vi "读取反控数据解析(子VI).vi"(6 "数据":string, 7 "命令编码CN":string) -> (2 "设置超时时间/min":i32=1, 3 "反控命令错误？":bool)   [LabVIEW 2016, in "数据传输系统-06.lvlib"]
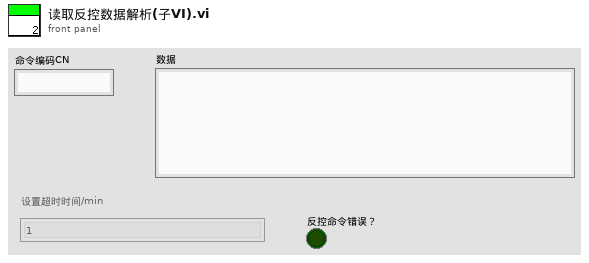
[diagram p1: front panel]
types:
  T1 = typedef "数据传输系统-06.lvlib/应用环境.ctl" = enum16{"STD", "GB212", "婉仪平台"}
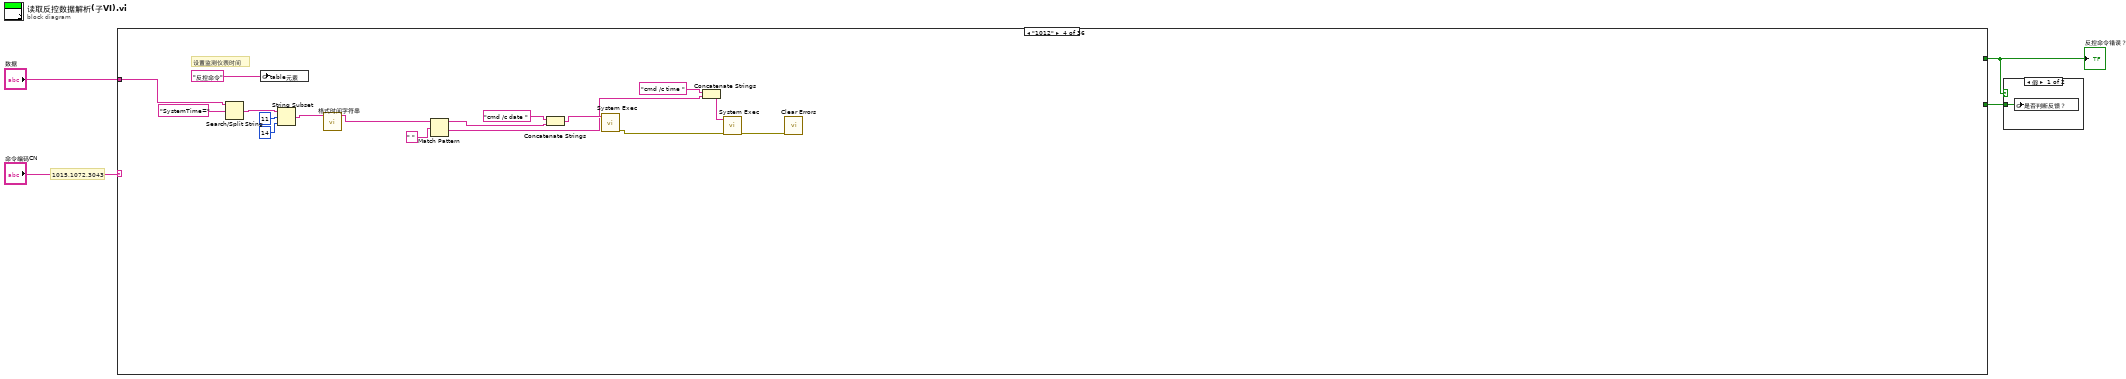
[diagram p0: block diagram]
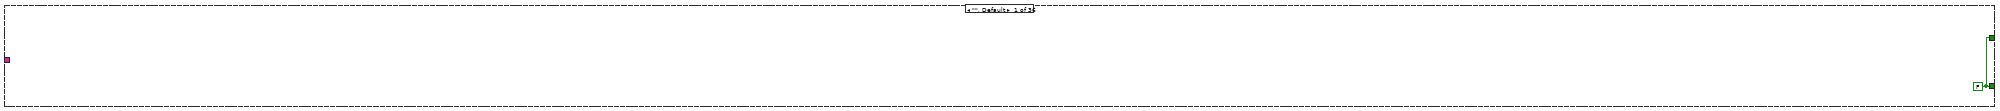
[diagram p2: hidden frame]
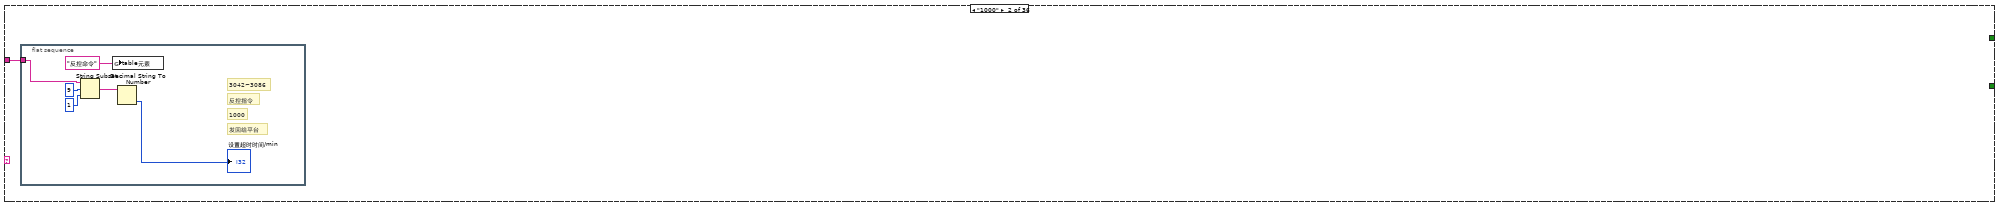
[diagram p3: hidden frame]
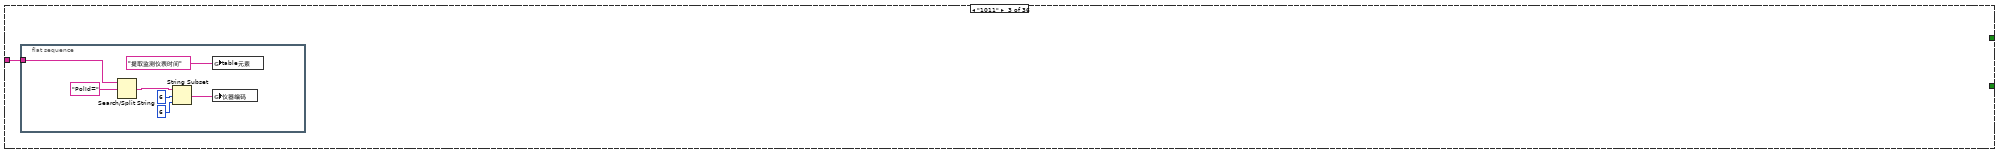
[diagram p4: hidden frame]
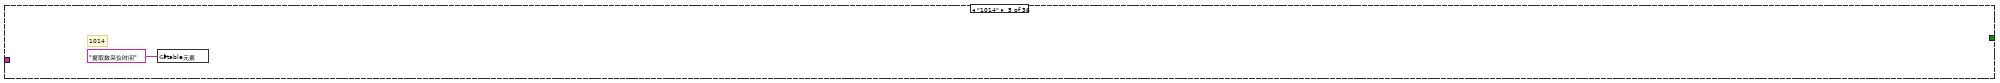
[diagram p5: hidden frame]
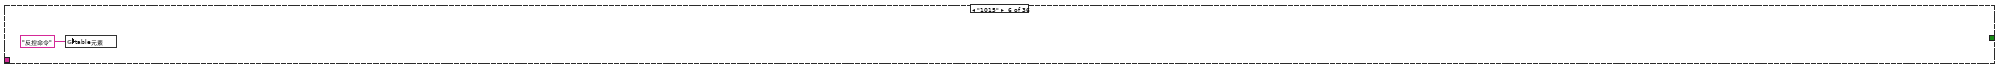
[diagram p6: hidden frame]
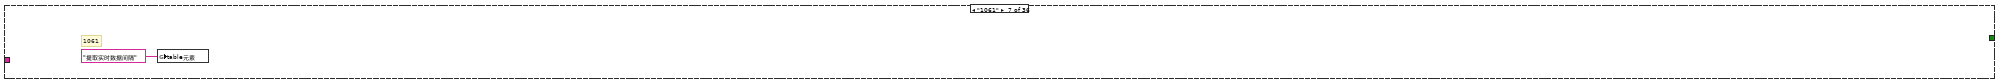
[diagram p7: hidden frame]
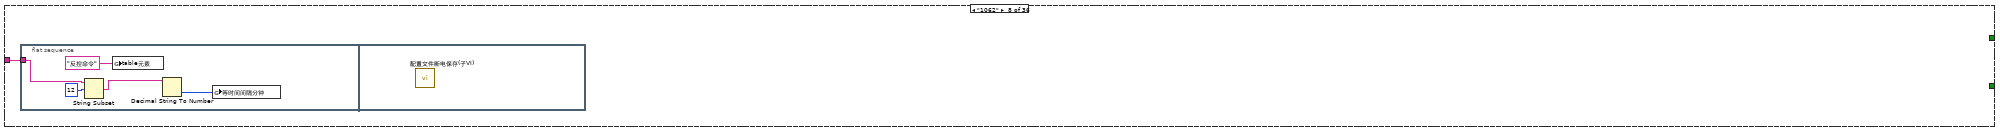
[diagram p8: hidden frame]
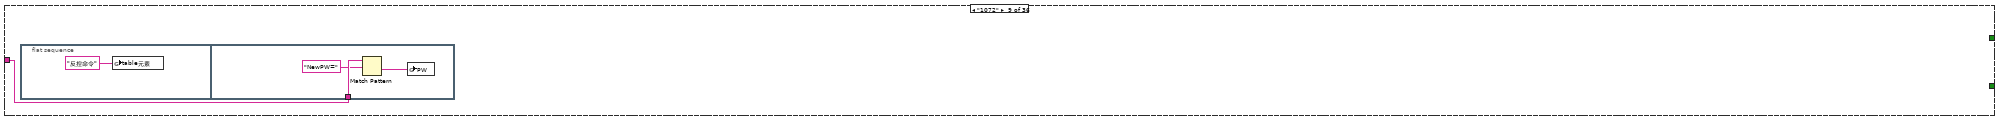
[diagram p9: hidden frame]
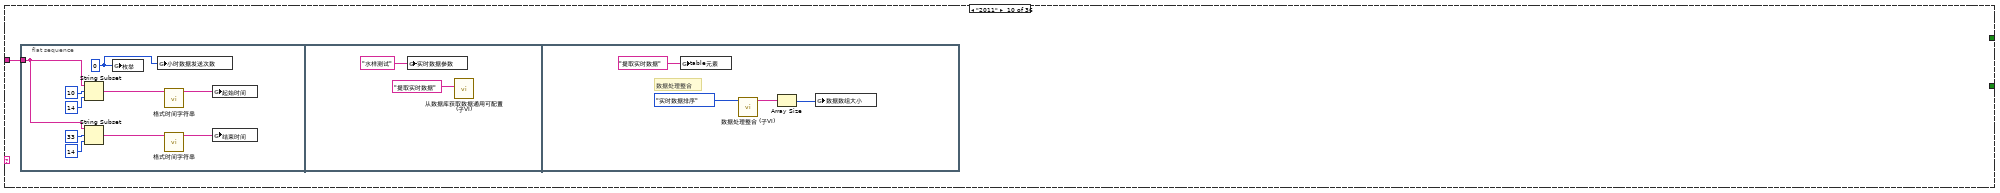
[diagram p10: hidden frame]
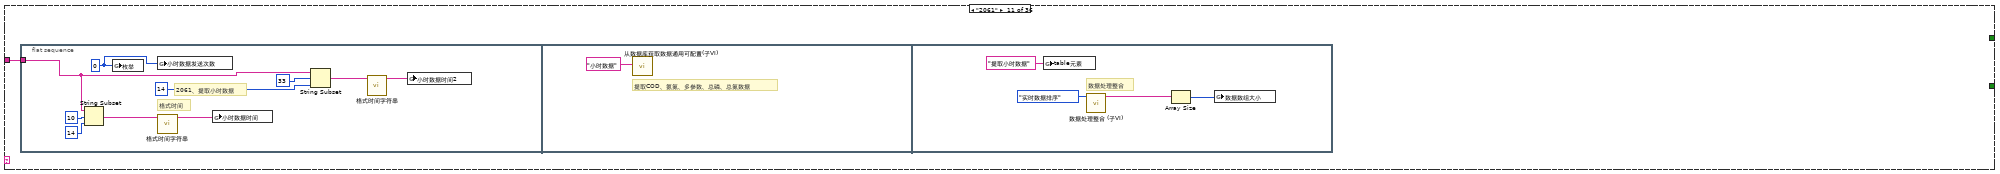
[diagram p11: hidden frame]
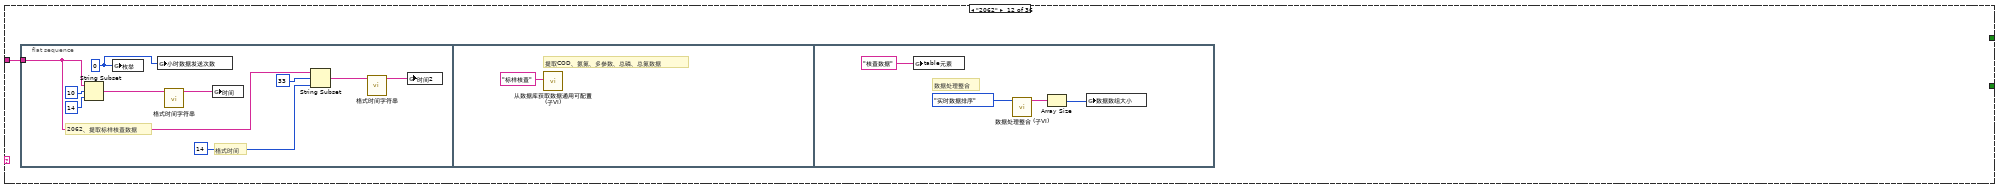
[diagram p12: hidden frame]
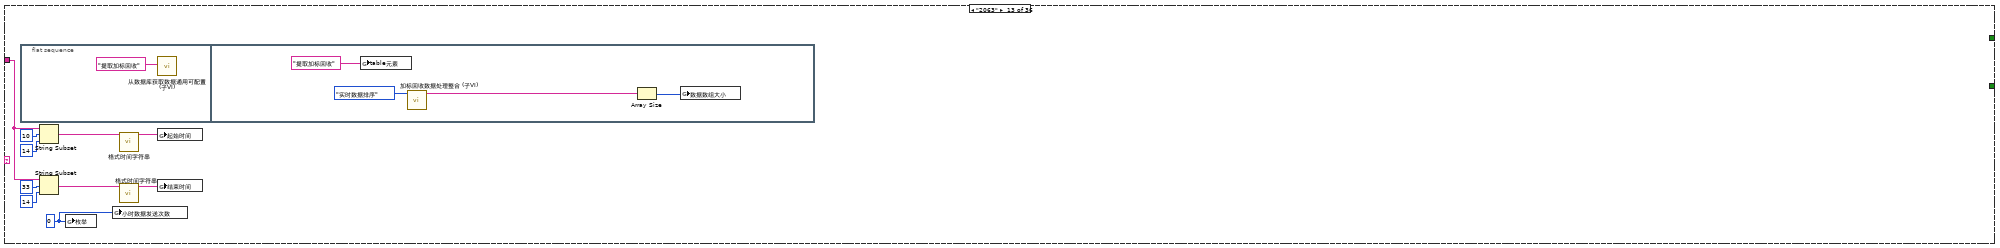
[diagram p13: hidden frame]
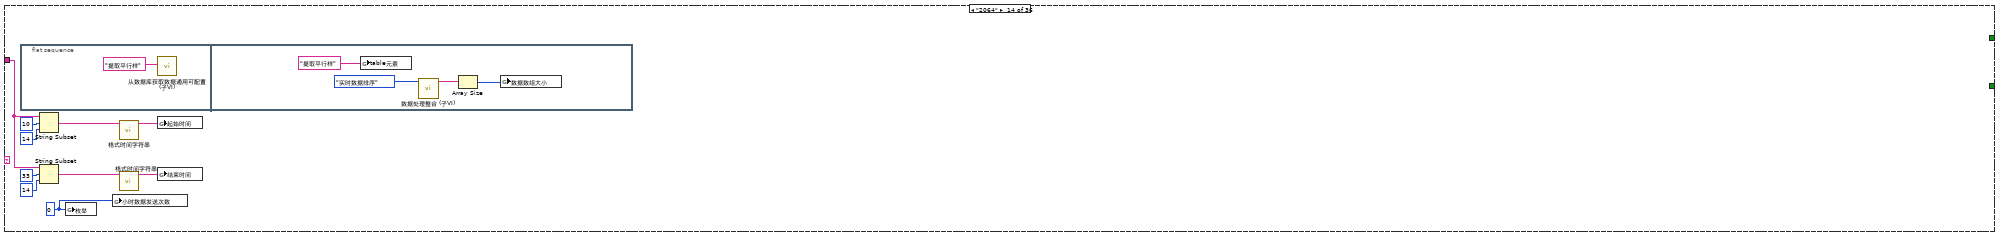
[diagram p14: hidden frame]
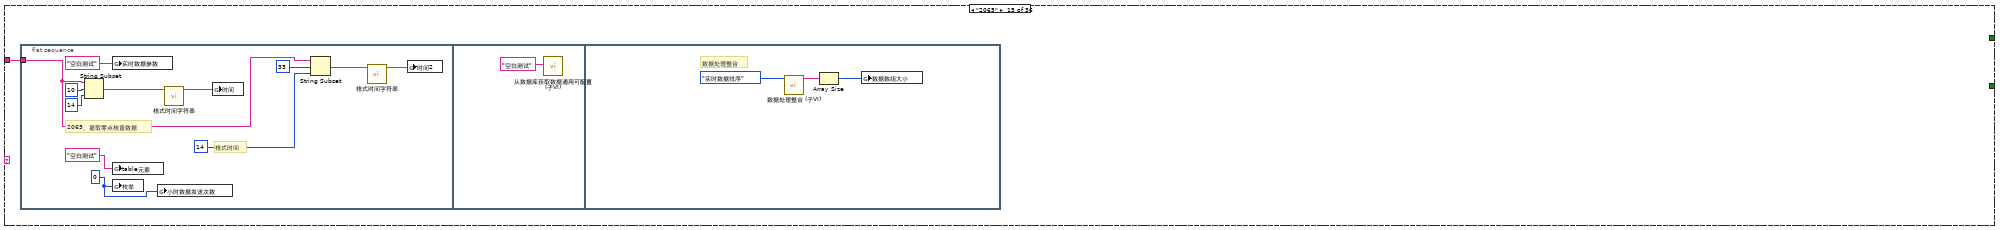
[diagram p15: hidden frame]
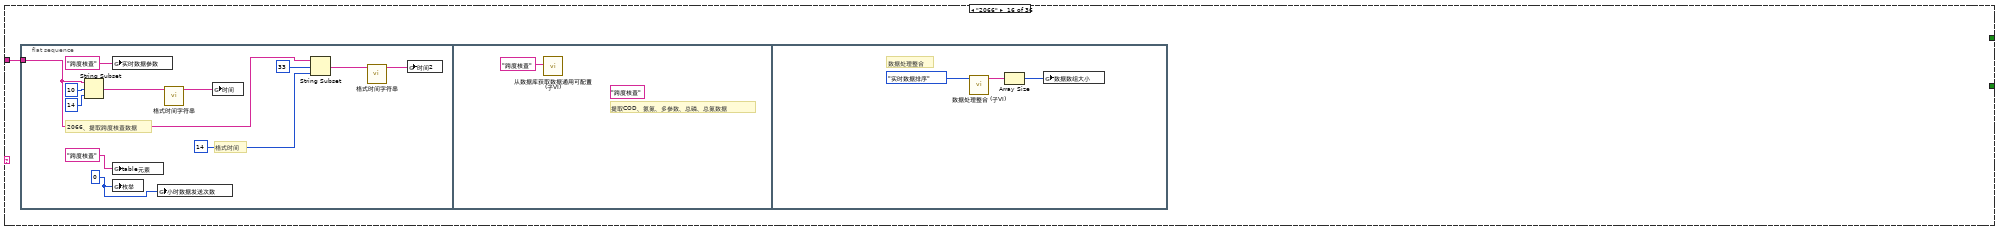
[diagram p16: hidden frame]
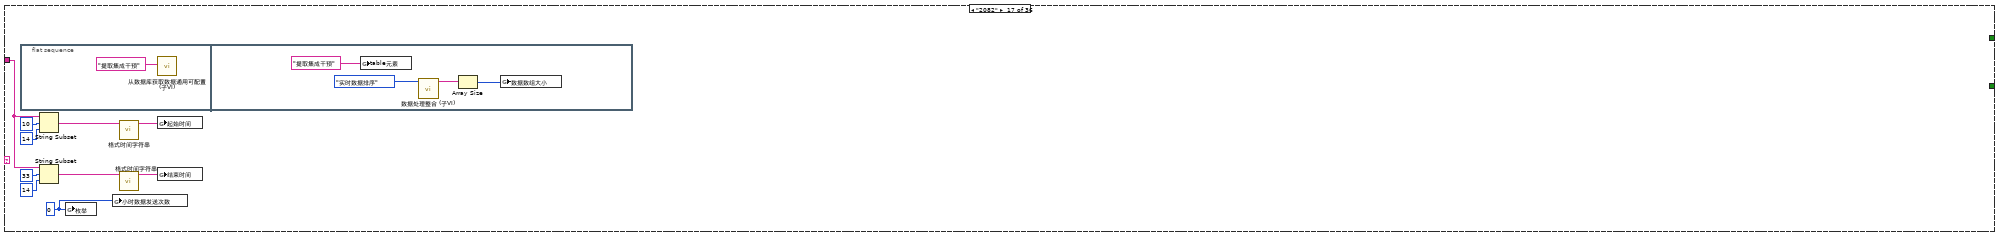
[diagram p17: hidden frame]
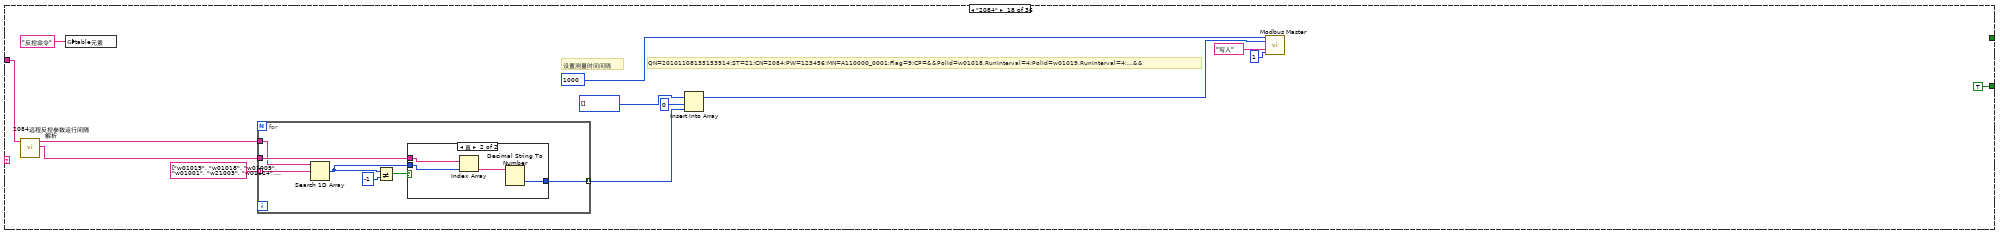
[diagram p18: hidden frame]
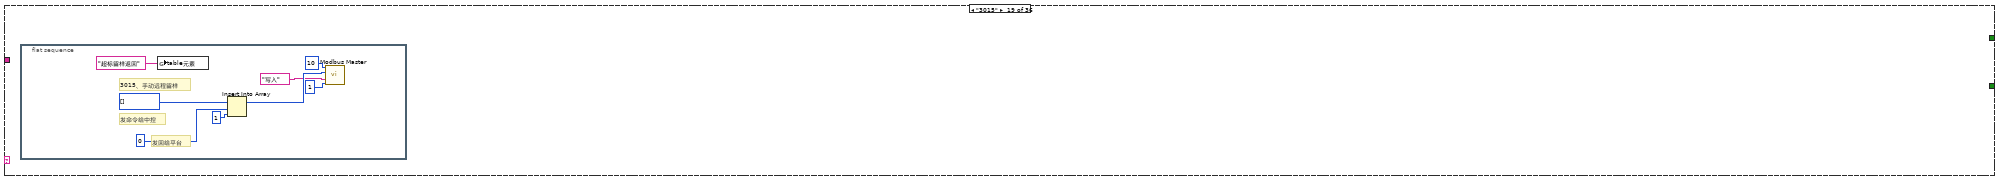
[diagram p20: hidden frame]
diagram:
  # "1015,1072,3043"
  n1 = case shown="\"1012\"" "命令编码CN" {
    selector: "命令编码CN" -> [_ _ _ _ _ _ _ _ _ _ _ _ _ _ _ _ _ _ _ _ _ _ _ _ _ _ _ _ _ w509 _ _ _ _ w649 _]
    tunnel: "数据" -> [_ w6 w13 w32 _ _ _ w41 w47 w52 w69 w85 w102 w116 w131 w148 w165 w191 _ w212 w368 _ _ w460 _ _ _ _ w508 w510 _ w571 w592 w613 w648 _]
    tunnel: [w5 _ _ _ _ _ _ _ _ _ _ _ _ _ _ _ _ _ _ _ _ _ _ _ _ _ _ _ _ _ _ _ _ _ _ _] -> w2
    tunnel: [w5 _ _ _ _ _ _ _ _ _ _ _ _ _ _ _ _ TRUE _ _ TRUE _ _ TRUE ("是否判断反馈？") _ _ _ _ _ TRUE _ _ _ _ _ _] -> w1
    frame "", Default {
      w5 = FALSE
    }
    frame "1000" {
      n2 = flat-sequence {
        tunnel: w6 -> [w8]
        frame #0 {
          # "发回给平台"
          # "3042~3086"
          # "反控指令"
          # "1000"
          n3 = String Subset(string=w8, offset (0)=9 ("偏移量(0)"), length (rest)=1 ("长度（剩余）")) -> (substring=w10:string)
          n4 = global write "全局1.vi" "table元素"("反控命令" ("新元素/子数组")) -> ()
          n5 = Decimal String To Number(string=w10) -> (number=→"设置超时时间/min":i32)  [unwired: 2 in, 1 out]
        }
      }
    }
    frame "1011" {
      n6 = flat-sequence {
        tunnel: w13 -> [w14]
        frame #0 {
          n7 = Search/Split String(string=w14, search string/char (-)="PolId=" ("搜索字符串/字符(-)")) -> (match + rest of string=w19:string)  [unwired: 1 in, 2 out]
          n8 = String Subset(string=w19, offset (0)=6 ("偏移量(0)"), length (rest)=6 ("长度（剩余）")) -> (substring=w16:string)
          n9 = global write "全局1.vi" "table元素"("提取监测仪表时间") -> ()
          n10 = global write "全局 提取仪器参数.vi" "仪器编码"(w16) -> ()
        }
      }
    }
    frame "1012" {
      # "设置监测仪表时间"
      n11 = Search/Split String(string=w32, search string/char (-)="SystemTime=" ("搜索字符串/字符(-)")) -> (match + rest of string=w35:string)  [unwired: 1 in, 2 out]
      n12 = global write "全局1.vi" "table元素"("反控命令" ("新元素/子数组")) -> ()
      n13 = String Subset(string=w35, offset (0)=11 ("偏移量(0)"), length (rest)=14 ("长度（剩余）")) -> (substring=w31:string)
      n14 = call "格式时间字符串.vi"("字符串"=w31) -> ("连接的字符串"=w29:string)  [unwired: 10 in]
      n15 = Match Pattern(string=w29, regular expression=" " ("子字符串;substring")) -> (before substring=w27:string, after substring=w23:string)  [unwired: 1 in, 2 out]
      n16 = Concatenate Strings("cmd /c date " ("command line"), w27) -> (w26:string)
      n17 = call <vilib>:"System Exec.vi"("command line"=w26) -> ("error out"=w25:errorcluster)  [unwired: 7 in, 3 out]
      n18 = Concatenate Strings("cmd /c time " ("command line"), w23) -> (w22:string)
      n19 = call <vilib>:"System Exec.vi"("error in (no error)"=w25, "command line"=w22) -> ("error out"=w21:errorcluster)  [unwired: 6 in, 3 out]
      n20 = call <vilib>:"Clear Errors.vi"("error in (no error)"=w21) -> ()  [unwired: 5 in, 2 out]
    }
    frame "1014" {
      # "1014"
      n21 = global write "全局1.vi" "table元素"("提取数采仪时间") -> ()
    }
    frame "1015" {
      n22 = global write "全局1.vi" "table元素"("反控命令" ("新元素/子数组")) -> ()
    }
    frame "1061" {
      # "1061"
      n23 = global write "全局1.vi" "table元素"("提取实时数据间隔") -> ()
    }
    frame "1062" {
      n24 = flat-sequence {
        tunnel: w41 -> [w44]
        frame #0 {
          n25 = String Subset(string=w44, offset (0)=12 ("偏移量(0)")) -> (substring=w45:string)  [unwired: 1 in]
          n26 = global write "全局1.vi" "table元素"("反控命令" ("新元素/子数组")) -> ()
          n27 = Decimal String To Number(string=w45) -> (number=w42:i32)  [unwired: 2 in, 1 out]
          n28 = global write "断电保存全局.vi" "等时间间隔分钟"(w42) -> ()
        }
        frame #1 {
          n29 = call "配置文件断电保存(子VI).vi"() -> ()  [unwired: 12 in]
        }
      }
    }
    frame "1072" {
      n30 = flat-sequence {
        tunnel: w47 -> [w51]
        frame #0 {
          n31 = global write "全局1.vi" "table元素"("反控命令" ("新元素/子数组")) -> ()
        }
        frame #1 {
          n32 = Match Pattern(string=w51, regular expression="NewPW=" ("正则表达式")) -> (after substring=w49:string)  [unwired: 1 in, 3 out]
          n33 = global write "断电保存全局.vi" "PW"(w49) -> ()
        }
      }
    }
    frame "2011" {
      n34 = flat-sequence {
        tunnel: w52 -> [w53]
        frame #0 {
          w58 = 0 ("数值")
          n35 = String Subset(string=w53, offset (0)=10 ("偏移量(0)"), length (rest)=14 ("长度（剩余）")) -> (substring=w61:string)
          n36 = String Subset(string=w53, offset (0)=33 ("偏移量(0)"), length (rest)=14 ("长度（剩余）")) -> (substring=w59:string)
          n37 = global write "全局1.vi" "枚举"(w58) -> ()
          n38 = global write "全局 小时数据发送次数.vi" "小时数据发送次数"(w58) -> ()
          n39 = call "格式时间字符串.vi"("字符串"=w61) -> ("连接的字符串"=w62:string)  [unwired: 10 in]
          n40 = call "格式时间字符串.vi"("字符串"=w59) -> ("连接的字符串"=w60:string)  [unwired: 10 in]
          n41 = global write "起始时间.vi" "起始时间"(w62) -> ()
          n42 = global write "起始时间.vi" "结束时间"(w60) -> ()
        }
        frame #1 {
          n43 = global write "全局 实时数据参数.vi" "实时数据参数"("水样测试") -> ()
          n44 = call "从数据库获取数据通用可配置(子VI).vi"("table输入"="提取实时数据" ("新元素/子数组")) -> ()  [unwired: 9 in, 2 out]
        }
        frame #2 {
          # "数据处理整合"
          n45 = global write "全局1.vi" "table元素"("提取实时数据" ("新元素/子数组")) -> ()
          n46 = call "数据处理整合 (子VI).vi"("枚举"=enum16{"实时数据排序", "小时数据排序"}."实时数据排序") -> ("已排序的数组"=w67:string[])  [unwired: 10 in]
          n47 = Array Size(array=w67) -> (size(s)=w68:i32)
          n48 = global write "全局 数据数组大小.vi" "数据数组大小"(w68) -> ()
        }
      }
    }
    frame "2061" {
      n49 = flat-sequence {
        tunnel: w69 -> [w70]
        frame #0 {
          w71 = 0 ("数值")
          # "格式时间"
          # "2061、提取小时数据"
          n50 = String Subset(string=w70, offset (0)=10 ("偏移量(0)"), length (rest)=14 ("长度（剩余）")) -> (substring=w74:string)
          n51 = global write "全局1.vi" "枚举"(w71) -> ()
          n52 = global write "全局 小时数据发送次数.vi" "小时数据发送次数"(w71) -> ()
          n53 = call "格式时间字符串.vi"("字符串"=w74) -> ("连接的字符串"=w75:string)  [unwired: 10 in]
          n54 = global write "全局 水样时间.vi" "小时数据时间"(w75) -> ()
          n55 = String Subset(string=w70, offset (0)=33 ("偏移量(0)"), length (rest)=14 ("长度（剩余）")) -> (substring=w73:string)
          n56 = call "格式时间字符串.vi"("字符串"=w73) -> ("连接的字符串"=w72:string)  [unwired: 10 in]
          n57 = global write "全局 时间2.vi" "小时数据时间2"(w72) -> ()
        }
        frame #1 {
          # "提取COD、氨氮、多参数、总磷、总氮数据"
          n58 = call "从数据库获取数据通用可配置(子VI).vi"("table输入"="小时数据" ("名称（未命名）")) -> ()  [unwired: 9 in, 2 out]
        }
        frame #2 {
          # "数据处理整合"
          n59 = global write "全局1.vi" "table元素"("提取小时数据" ("新元素/子数组")) -> ()
          n60 = call "数据处理整合 (子VI).vi"("枚举"=enum16{"实时数据排序", "小时数据排序"}."实时数据排序") -> ("已排序的数组"=w84:string[])  [unwired: 10 in]
          n61 = Array Size(array=w84) -> (size(s)=w83:i32)
          n62 = global write "全局 数据数组大小.vi" "数据数组大小"(w83) -> ()
        }
      }
    }
    frame "2062" {
      n63 = flat-sequence {
        tunnel: w85 -> [w86]
        frame #0 {
          w87 = 0 ("数值")
          # "格式时间"
          # "2062、提取标样核查数据"
          n64 = String Subset(string=w86, offset (0)=10 ("偏移量(0)"), length (rest)=14 ("长度（剩余）")) -> (substring=w90:string)
          n65 = global write "全局1.vi" "枚举"(w87) -> ()
          n66 = global write "全局 小时数据发送次数.vi" "小时数据发送次数"(w87) -> ()
          n67 = call "格式时间字符串.vi"("字符串"=w90) -> ("连接的字符串"=w91:string)  [unwired: 10 in]
          n68 = global write "全局 水样时间.vi" "时间"(w91) -> ()
          n69 = String Subset(string=w86, offset (0)=33 ("偏移量(0)"), length (rest)=14 ("长度（剩余）")) -> (substring=w89:string)
          n70 = call "格式时间字符串.vi"("字符串"=w89) -> ("连接的字符串"=w88:string)  [unwired: 10 in]
          n71 = global write "全局 时间2.vi" "时间2"(w88) -> ()
        }
        frame #1 {
          # "提取COD、氨氮、多参数、总磷、总氮数据"
          n72 = call "从数据库获取数据通用可配置(子VI).vi"("table输入"="标样核查" ("新元素/子数组")) -> ()  [unwired: 9 in, 2 out]
        }
        frame #2 {
          # "数据处理整合"
          n73 = global write "全局1.vi" "table元素"("核查数据" ("新元素/子数组")) -> ()
          n74 = call "数据处理整合 (子VI).vi"("枚举"=enum16{"实时数据排序", "小时数据排序"}."实时数据排序") -> ("已排序的数组"=w99:string[])  [unwired: 10 in]
          n75 = Array Size(array=w99) -> (size(s)=w100:i32)
          n76 = global write "全局 数据数组大小.vi" "数据数组大小"(w100) -> ()
        }
      }
    }
    frame "2063" {
      w101 = 0 ("数值")
      n77 = flat-sequence {
        frame #0 {
          n78 = call "从数据库获取数据通用可配置(子VI).vi"("table输入"="提取加标回收" ("新元素/子数组")) -> ()  [unwired: 9 in, 2 out]
        }
        frame #1 {
          n79 = global write "全局1.vi" "table元素"("提取加标回收" ("新元素/子数组")) -> ()
          n80 = call "加标回收数据处理整合 (子VI).vi"("枚举"=enum16{"实时数据排序", "小时数据排序"}."实时数据排序") -> ("已排序的数组"=w113:string[])  [unwired: 10 in]
          n81 = Array Size(array=w113) -> (size(s)=w115:i32)
          n82 = global write "全局 数据数组大小.vi" "数据数组大小"(w115) -> ()
        }
      }
      n83 = String Subset(string=w102, offset (0)=10 ("偏移量(0)"), length (rest)=14 ("长度（剩余）")) -> (substring=w104:string)
      n84 = String Subset(string=w102, offset (0)=33 ("偏移量(0)"), length (rest)=14 ("长度（剩余）")) -> (substring=w106:string)
      n85 = global write "全局1.vi" "枚举"(w101) -> ()
      n86 = global write "全局 小时数据发送次数.vi" "小时数据发送次数"(w101) -> ()
      n87 = call "格式时间字符串.vi"("字符串"=w104) -> ("连接的字符串"=w103:string)  [unwired: 10 in]
      n88 = call "格式时间字符串.vi"("字符串"=w106) -> ("连接的字符串"=w105:string)  [unwired: 10 in]
      n89 = global write "起始时间.vi" "起始时间"(w103) -> ()
      n90 = global write "起始时间.vi" "结束时间"(w105) -> ()
    }
    frame "2064" {
      w121 = 0 ("数值")
      n91 = flat-sequence {
        frame #0 {
          n92 = call "从数据库获取数据通用可配置(子VI).vi"("table输入"="提取平行样" ("新元素/子数组")) -> ()  [unwired: 9 in, 2 out]
        }
        frame #1 {
          n93 = global write "全局1.vi" "table元素"("提取平行样" ("新元素/子数组")) -> ()
          n94 = call "数据处理整合 (子VI).vi"("枚举"=enum16{"实时数据排序", "小时数据排序"}."实时数据排序") -> ("已排序的数组"=w130:string[])  [unwired: 10 in]
          n95 = Array Size(array=w130) -> (size(s)=w129:i32)
          n96 = global write "全局 数据数组大小.vi" "数据数组大小"(w129) -> ()
        }
      }
      n97 = String Subset(string=w116, offset (0)=10 ("偏移量(0)"), length (rest)=14 ("长度（剩余）")) -> (substring=w124:string)
      n98 = String Subset(string=w116, offset (0)=33 ("偏移量(0)"), length (rest)=14 ("长度（剩余）")) -> (substring=w122:string)
      n99 = global write "全局1.vi" "枚举"(w121) -> ()
      n100 = global write "全局 小时数据发送次数.vi" "小时数据发送次数"(w121) -> ()
      n101 = call "格式时间字符串.vi"("字符串"=w124) -> ("连接的字符串"=w125:string)  [unwired: 10 in]
      n102 = call "格式时间字符串.vi"("字符串"=w122) -> ("连接的字符串"=w123:string)  [unwired: 10 in]
      n103 = global write "起始时间.vi" "起始时间"(w125) -> ()
      n104 = global write "起始时间.vi" "结束时间"(w123) -> ()
    }
    frame "2065" {
      n105 = flat-sequence {
        tunnel: w131 -> [w133]
        frame #0 {
          w134 = 0 ("数值")
          # "格式时间"
          # "2065、提取零点核查数据"
          n106 = String Subset(string=w133, offset (0)=10 ("偏移量(0)"), length (rest)=14 ("长度（剩余）")) -> (substring=w138:string)
          n107 = global write "全局 实时数据参数.vi" "实时数据参数"("空白测试" ("新元素/子数组")) -> ()
          n108 = global write "全局1.vi" "table元素"("空白测试" ("新元素/子数组")) -> ()
          n109 = global write "全局1.vi" "枚举"(w134) -> ()
          n110 = global write "全局 小时数据发送次数.vi" "小时数据发送次数"(w134) -> ()
          n111 = call "格式时间字符串.vi"("字符串"=w138) -> ("连接的字符串"=w139:string)  [unwired: 10 in]
          n112 = global write "全局 水样时间.vi" "时间"(w139) -> ()
          n113 = String Subset(string=w133, offset (0)=33 ("偏移量(0)"), length (rest)=14 ("长度（剩余）")) -> (substring=w137:string)
          n114 = call "格式时间字符串.vi"("字符串"=w137) -> ("连接的字符串"=w136:string)  [unwired: 10 in]
          n115 = global write "全局 时间2.vi" "时间2"(w136) -> ()
        }
        frame #1 {
          n116 = call "从数据库获取数据通用可配置(子VI).vi"("table输入"="空白测试" ("新元素/子数组")) -> ()  [unwired: 9 in, 2 out]
        }
        frame #2 {
          # "数据处理整合"
          n117 = call "数据处理整合 (子VI).vi"("枚举"=enum16{"实时数据排序", "小时数据排序"}."实时数据排序") -> ("已排序的数组"=w146:string[])  [unwired: 10 in]
          n118 = Array Size(array=w146) -> (size(s)=w147:i32)
          n119 = global write "全局 数据数组大小.vi" "数据数组大小"(w147) -> ()
        }
      }
    }
    frame "2066" {
      n120 = flat-sequence {
        tunnel: w148 -> [w150]
        frame #0 {
          w151 = 0 ("数值")
          # "格式时间"
          # "2066、提取跨度核查数据"
          n121 = String Subset(string=w150, offset (0)=10 ("偏移量(0)"), length (rest)=14 ("长度（剩余）")) -> (substring=w155:string)
          n122 = global write "全局 实时数据参数.vi" "实时数据参数"("跨度核查" ("新元素/子数组")) -> ()
          n123 = global write "全局1.vi" "table元素"("跨度核查" ("新元素/子数组")) -> ()
          n124 = global write "全局1.vi" "枚举"(w151) -> ()
          n125 = global write "全局 小时数据发送次数.vi" "小时数据发送次数"(w151) -> ()
          n126 = call "格式时间字符串.vi"("字符串"=w155) -> ("连接的字符串"=w156:string)  [unwired: 10 in]
          n127 = global write "全局 水样时间.vi" "时间"(w156) -> ()
          n128 = String Subset(string=w150, offset (0)=33 ("偏移量(0)"), length (rest)=14 ("长度（剩余）")) -> (substring=w154:string)
          n129 = call "格式时间字符串.vi"("字符串"=w154) -> ("连接的字符串"=w153:string)  [unwired: 10 in]
          n130 = global write "全局 时间2.vi" "时间2"(w153) -> ()
        }
        frame #1 {
          (unwired) "跨度核查" ("名称（未命名）")
          # "提取COD、氨氮、多参数、总磷、总氮数据"
          n131 = call "从数据库获取数据通用可配置(子VI).vi"("table输入"="跨度核查" ("新元素/子数组")) -> ()  [unwired: 9 in, 2 out]
        }
        frame #2 {
          # "数据处理整合"
          n132 = call "数据处理整合 (子VI).vi"("枚举"=enum16{"实时数据排序", "小时数据排序"}."实时数据排序") -> ("已排序的数组"=w164:string[])  [unwired: 10 in]
          n133 = Array Size(array=w164) -> (size(s)=w163:i32)
          n134 = global write "全局 数据数组大小.vi" "数据数组大小"(w163) -> ()
        }
      }
    }
    frame "2082" {
      w170 = 0 ("数值")
      n135 = flat-sequence {
        frame #0 {
          n136 = call "从数据库获取数据通用可配置(子VI).vi"("table输入"="提取集成干预" ("新元素/子数组")) -> ()  [unwired: 9 in, 2 out]
        }
        frame #1 {
          n137 = global write "全局1.vi" "table元素"("提取集成干预" ("新元素/子数组")) -> ()
          n138 = call "数据处理整合 (子VI).vi"("枚举"=enum16{"实时数据排序", "小时数据排序"}."实时数据排序") -> ("已排序的数组"=w179:string[])  [unwired: 10 in]
          n139 = Array Size(array=w179) -> (size(s)=w178:i32)
          n140 = global write "全局 数据数组大小.vi" "数据数组大小"(w178) -> ()
        }
      }
      n141 = String Subset(string=w165, offset (0)=10 ("偏移量(0)"), length (rest)=14 ("长度（剩余）")) -> (substring=w173:string)
      n142 = String Subset(string=w165, offset (0)=33 ("偏移量(0)"), length (rest)=14 ("长度（剩余）")) -> (substring=w171:string)
      n143 = global write "全局1.vi" "枚举"(w170) -> ()
      n144 = global write "全局 小时数据发送次数.vi" "小时数据发送次数"(w170) -> ()
      n145 = call "格式时间字符串.vi"("字符串"=w173) -> ("连接的字符串"=w174:string)  [unwired: 10 in]
      n146 = call "格式时间字符串.vi"("字符串"=w171) -> ("连接的字符串"=w172:string)  [unwired: 10 in]
      n147 = global write "起始时间.vi" "起始时间"(w174) -> ()
      n148 = global write "起始时间.vi" "结束时间"(w172) -> ()
    }
    frame "2084" {
      # "设置测量时间间隔"
      # "QN=20101108135153914;ST=21;CN=2084;PW=123456;MN=A110000_0001;Flag=9;CP=&&PolId=w01018,RunInterval=4;PolId=w01019,RunInterval=4;...&&"
      n149 = call "2084远程反控参数运行间隔解析.vi"("字符串"=w191) -> ("Value"=w182:string[], "因子编码"=w183:string[])  [unwired: 9 in]
      n150 = global write "全局1.vi" "table元素"("反控命令" ("新元素/子数组")) -> ()
      n151 = for {
        tunnel: w183 -> [w198]
        tunnel: w182 -> [w199]
        tunnel: string[] ["w01019", "w01018", "w01009", "w01001", "w21003", "w01014", "w01010", "w01003", "w21001", "w21011", "w01016", "w19011", "w21006", "w21019", "w01100", "w20120", "w20115", "w20122", "w20123", "w20121", "w20124", "w20111"] ("因子编码") -> [w197] mode=indexing
        tunnel: [w193] -> w181 mode=indexing
        n152 = Search 1D Array(1D array=w198, element=w197) -> (index of element=w194:i32)  [unwired: 1 in]
        n153 = Not Equal?(x=w194, y=-1) -> (x != y?=w195:bool)
        n154 = case shown="真" w195 {
          tunnel: w199 -> [_ w203]
          tunnel: w194 -> [_ w202]
          tunnel: [_ w200] -> w193
          frame False {
          }
          frame True {
            n155 = Index Array(array=w203, index=w202) -> (element=w201:string)
            n156 = Decimal String To Number(string=w201) -> (number=w200:i32)  [unwired: 2 in, 1 out]
          }
        }
      }
      n157 = Insert Into Array(array=u16[] [] ("holding register values"), index=0 ("索引"), new element=w181) -> (w187:u16[])
      n158 = call "Modbus Master.vi"("starting address"=u16 1000, "holding register values"=w187, "读取写入选择"="写入", "Unit ID"=u8 1) -> ()  [unwired: 5 in, 7 out]
    }
    frame "3015" {
      n159 = flat-sequence {
        frame #0 {
          # "发命令给中控"
          # "发回给平台"
          # "3015、手动远程留样"
          n160 = global write "全局1.vi" "table元素"("超标留样返回" ("新元素/子数组")) -> ()
          n161 = Insert Into Array(array=u16[] [] ("holding register values"), index=0 ("索引"), new element=u16 1 ("新元素/子数组")) -> (w207:u16[])
          n162 = call "Modbus Master.vi"("starting address"=u16 10, "holding register values"=w207, "读取写入选择"="写入", "Unit ID"=u8 1) -> ()  [unwired: 5 in, 7 out]
        }
      }
    }
    frame "3020" {
      n163 = flat-sequence {
        tunnel: [w224] -> w218
        tunnel: [w225] -> w217
        tunnel: [w221] -> w216
        tunnel: [w223] -> w215
        tunnel: w212 -> [w222]
        tunnel: [w222] -> w214
        tunnel: w218 -> [w253]
        tunnel: w217 -> [w254]
        tunnel: w216 -> [w255]
        tunnel: w215 -> [w257]
        tunnel: [w256] -> w213
        tunnel: w214 -> [w256]
        tunnel: w213 -> [w340]
        frame #0 {
          w219 = "操作日志报警信息" ("名称（未命名）")
          w228 = 0 ("数值")
          # "3020、提取日志、报警，仪器参数"
          n164 = call "日志报警参数选择 (子VI).vi"("String输入"=w222) -> ("输出boll数组"=w220:bool[], "输出char数组"=w221:string[])  [unwired: 7 in, 2 out]
          n165 = global write "全局1.vi" "枚举"(w228) -> ()
          n166 = global write "全局 小时数据发送次数.vi" "小时数据发送次数"(w228) -> ()
          n167 = Search/Split String(string=w222, search string/char (-)="BeginTime=" ("搜索字符串")) -> (match + rest of string=w227:string)  [unwired: 1 in, 2 out]
          n168 = case shown="\"\"" w227 {
            tunnel: ["1904/01/01 00:00:00" w250] -> w230
            tunnel: w227 -> [_ w244]
            tunnel: [w238 w245] -> w226
            frame "" {
              n169 = Get Date/Time In Seconds() -> (seconds since 1Jan1904=w240:timestamp)
              n170 = Format Date/Time String(time format string (%c)="%Y/%m/%d %H:%M:%S" ("时间格式字符串(%c)"), seconds (now)=w240) -> (date/time string=w241:string)  [unwired: 1 in]
              n171 = Search and Replace String(input string=w241, search string="." ("搜索字符串")) -> (result string=w238:string)  [unwired: 6 in, 3 out]
            }
            frame "真", Default {
              # "格式时间"
              n172 = String Subset(string=w244, offset (0)=10 ("偏移量(0)"), length (rest)=14 ("长度（剩余）")) -> (substring=w249:string)
              n173 = String Subset(string=w244, offset (0)=33 ("偏移量(0)"), length (rest)=14 ("长度（剩余）")) -> (substring=w248:string)
              n174 = call "格式时间字符串.vi"("字符串"=w249) -> ("连接的字符串"=w250:string)  [unwired: 10 in]
              n175 = call "格式时间字符串.vi"("字符串"=w248) -> ("连接的字符串"=w245:string)  [unwired: 10 in]
            }
          }
          n176 = Or Array Elements(Boolean array=w220) -> (logical OR=w223:bool)
          n177 = Obtain Queue(name (unnamed)=w219, element data type=w219) -> (queue out=w224:refnum<queue>, error out=w225:errorcluster)  [unwired: 3 in, 1 out]
          n178 = case shown="真" w223 {
            tunnel: w224 -> [_ w232]
            tunnel: w220 -> [_ w231]
            frame False {
            }
            frame True {
              n179 = for {
                tunnel: w231 -> [w234] mode=indexing
                tunnel: w232 -> [w233]
                i -> [w235]
                n180 = case shown="真" w234 {
                  tunnel: w235 -> [_ w237]
                  tunnel: w233 -> [_ w236]
                  frame False {
                  }
                  frame True {
                    n181 = call "提取日志报警参数入列队 (子VI).vi"("索引"=w237, "队列输入"=w236) -> ()  [unwired: 10 in]
                  }
                }
              }
            }
          }
          n182 = global write "全局 水样时间.vi" "时间"(w230) -> ()
          n183 = global write "全局 时间2.vi" "时间2"(w226) -> ()
        }
        frame #1 {
          # "按需求提取COD、氨氮、总磷、总氮日志"
          # "按需求提取COD、氨氮、总磷、总氮日志"
          n184 = case shown="真" w257 {
            tunnel: w254 -> [_ w260]
            tunnel: w253 -> [_ w259]
            tunnel: w255 -> [_ w258]
            frame False {
            }
            frame True {
              n185 = while {
                shift-right: [w261] -> _
                shift-left: w259 -> [w268]
                tunnel: w260 -> [w267]
                tunnel: w258 -> [w262]
                stop <- w264 stop-if-true
                n186 = Dequeue Element(queue=w268, error in (no error)=w267) -> (queue out=w266:refnum<queue>, element=w263:string)  [unwired: 1 in, 2 out]
                n187 = case shown="\"CODMn\", 默认" w263 {
                  tunnel: w266 -> [_ _ _ _ _ _ _ _ _ _ _ _ _ _]
                  tunnel: w262 -> [w270 w275 w280 w285 w290 w296 w299 w304 w309 w314 w319 w324 w329 w334]
                  frame "CODMn", Default {
                    n188 = Index Array(array=w270, index=0 ("索引")) -> (element=w269:string)
                    n189 = call "数据表比对.vi"("仪器日志参数"="CODMn" ("元素"), "table输入"=w269) -> ("待发送数据"=w272:string[][])  [unwired: 6 in, 3 out]
                    n190 = global write "全局 所有参数.vi" "CODMn"(w272) -> ()
                  }
                  frame "CODCr" {
                    n191 = Index Array(array=w275, index=1 ("索引")) -> (element=w274:string)
                    n192 = call "数据表比对.vi"("仪器日志参数"="CODCr" ("元素"), "table输入"=w274) -> ("待发送数据"=w277:string[][])  [unwired: 6 in, 3 out]
                    n193 = global write "全局 所有参数.vi" "CODCr"(w277) -> ()
                  }
                  frame "氨氮" {
                    n194 = Index Array(array=w280, index=2 ("索引")) -> (element=w279:string)
                    n195 = call "数据表比对.vi"("仪器日志参数"="氨氮" ("元素"), "table输入"=w279) -> ("待发送数据"=w282:string[][])  [unwired: 6 in, 3 out]
                    n196 = global write "全局 所有参数.vi" "氨氮"(w282) -> ()
                  }
                  frame "总磷" {
                    n197 = Index Array(array=w285, index=3 ("索引")) -> (element=w284:string)
                    n198 = call "数据表比对.vi"("仪器日志参数"="总磷" ("元素"), "table输入"=w284) -> ("待发送数据"=w287:string[][])  [unwired: 6 in, 3 out]
                    n199 = global write "全局 所有参数.vi" "总磷"(w287) -> ()
                  }
                  frame "总氮" {
                    n200 = Index Array(array=w290, index=4 ("索引")) -> (element=w289:string)
                    n201 = call "数据表比对.vi"("仪器日志参数"="总氮" ("元素"), "table输入"=w289) -> ("待发送数据"=w292:string[][])  [unwired: 6 in, 3 out]
                    n202 = global write "全局 所有参数.vi" "总氮"(w292) -> ()
                  }
                  frame "数采仪" {
                    n203 = Index Array(array=w296, index=5 ("索引")) -> (element=w294:string)
                    n204 = call "数据表比对.vi"("仪器日志参数"="系统" ("元素"), "table输入"=w294) -> ("待发送数据"=w297:string[][])  [unwired: 6 in, 3 out]
                    n205 = global write "全局 所有参数.vi" "DO"(w297) -> ()
                  }
                  frame "PH" {
                    n206 = Index Array(array=w299, index=6 ("索引")) -> (element=w300:string)
                    n207 = call "数据表比对.vi"("仪器日志参数"="PH" ("元素"), "table输入"=w300) -> ("待发送数据"=w302:string[][])  [unwired: 6 in, 3 out]
                    n208 = global write "全局 所有参数.vi" "PH"(w302) -> ()
                  }
                  frame "电导率" {
                    n209 = Index Array(array=w304, index=7 ("索引")) -> (element=w305:string)
                    n210 = call "数据表比对.vi"("仪器日志参数"="电导率" ("元素"), "table输入"=w305) -> ("待发送数据"=w307:string[][])  [unwired: 6 in, 3 out]
                    n211 = global write "全局 所有参数.vi" "电导率"(w307) -> ()
                  }
                  frame "水温" {
                    n212 = Index Array(array=w309, index=8 ("索引")) -> (element=w310:string)
                    n213 = call "数据表比对.vi"("仪器日志参数"="水温" ("元素"), "table输入"=w310) -> ("待发送数据"=w312:string[][])  [unwired: 6 in, 3 out]
                    n214 = global write "全局 所有参数.vi" "水温"(w312) -> ()
                  }
                  frame "DO" {
                    n215 = Index Array(array=w314, index=9 ("索引")) -> (element=w315:string)
                    n216 = call "数据表比对.vi"("仪器日志参数"="溶解氧" ("元素"), "table输入"=w315) -> ("待发送数据"=w317:string[][])  [unwired: 6 in, 3 out]
                    n217 = global write "全局 所有参数.vi" "DO"(w317) -> ()
                  }
                  frame "浊度" {
                    n218 = Index Array(array=w319, index=10 ("索引")) -> (element=w320:string)
                    n219 = call "数据表比对.vi"("仪器日志参数"="浊度" ("元素"), "table输入"=w320) -> ("待发送数据"=w322:string[][])  [unwired: 6 in, 3 out]
                    n220 = global write "全局 所有参数.vi" "浊度"(w322) -> ()
                  }
                  frame "叶绿素" {
                    n221 = Index Array(array=w324, index=11 ("索引")) -> (element=w325:string)
                    n222 = call "数据表比对.vi"("仪器日志参数"="叶绿素" ("元素"), "table输入"=w325) -> ("待发送数据"=w327:string[][])  [unwired: 6 in, 3 out]
                    n223 = global write "全局 所有参数.vi" "叶绿素"(w327) -> ()
                  }
                  frame "藻密度" {
                    n224 = Index Array(array=w329, index=12 ("索引")) -> (element=w330:string)
                    n225 = call "数据表比对.vi"("仪器日志参数"="藻密度" ("元素"), "table输入"=w330) -> ("待发送数据"=w332:string[][])  [unwired: 6 in, 3 out]
                    n226 = global write "全局 所有参数.vi" "藻密度"(w332) -> ()
                  }
                  frame "ORP" {
                    n227 = Index Array(array=w334, index=13 ("索引")) -> (element=w335:string)
                    n228 = call "数据表比对.vi"("仪器日志参数"="ORP" ("元素"), "table输入"=w335) -> ("待发送数据"=w337:string[][])  [unwired: 6 in, 3 out]
                    n229 = global write "全局 所有参数.vi" "ORP"(w337) -> ()
                  }
                }
                n230 = Get Queue Status(queue=w266) -> (queue out=w261:refnum<queue>, # elements in queue=w265:i32)  [unwired: 2 in, 6 out]
                n231 = Equal To 0?(x=w265) -> (x = 0?=w264:bool)
              }
            }
          }
        }
        frame #2 {
          w349 = "InfoId=" ("搜索字符串/字符(-)")
          n232 = Spreadsheet String To Array(delimiter (Tab)=";" ("分隔符(Tab)"), format string="" ("格式字符串"), spreadsheet string=w340, array type (2D Dbl)=string[] []) -> (array=w341:string[])
          n233 = Index Array(array=w341) -> (element=w339:string)  [unwired: 1 in]
          n234 = Search/Split String(string=w339, search string/char (-)=w349) -> (match + rest of string=w348:string)  [unwired: 1 in, 2 out]
          n235 = Search and Replace String(replace all?=TRUE ("替换全部？(F)"), input string=w348, search string=w349, replace string="" ("替换字符串(\"\")")) -> (result string=w345:string)  [unwired: 4 in, 3 out]
          n236 = Spreadsheet String To Array(delimiter (Tab)="," ("分隔符(Tab)"), format string="" ("格式字符串"), spreadsheet string=w345, array type (2D Dbl)=string[] []) -> (array=w347:string[])
          n237 = Index Array(array=w347) -> (element=w346:string)  [unwired: 1 in]
          n238 = case shown="\"i12001\"" w346 {
            tunnel: ["操作日志" ("名称（未命名）") "提取仪器参数" ("名称（未命名）") "报警信息" ("名称（未命名）") "" ("名称（未命名）")] -> w355
            tunnel: [w357 1 ("数据数组大小") 1 _] -> w356
            tunnel: w345 -> [_ w361 _ _]
            frame "i11001", "i21001" {
              # "数据处理整合"
              # "i11001日志"
              n239 = call "数据处理整合 (子VI).vi"("枚举"=enum16{"实时数据排序", "小时数据排序"}."实时数据排序") -> ("已排序的数组"=w358:string[])  [unwired: 10 in]
              n240 = Array Size(array=w358) -> (size(s)=w357:i32)
            }
            frame "i13001", "i13002", "i13003", "i13004", "i13005", "i13006", "i13007", "i13008", "i13009", "i13010", "i13011", "i13012", "i13013", "i13014", "i13015", "i13016", "i13017", "i13101", "i13102", "i13103", "i13104", "i13105", "i13106", "i13107", "i13108", "i13109", "i13110" {
              n241 = call "数据处理直接插入整合 (子VI).vi"() -> ()  [unwired: 12 in]
              n242 = global write "全局 提取仪器参数.vi" "参数编码"(w361) -> ()
            }
            frame "i12001" {
              # "i12001状态"
              n243 = call "数据处理直接插入整合 (子VI).vi"() -> ()  [unwired: 12 in]
            }
            frame Default {
            }
          }
          n244 = global write "全局1.vi" "table元素"(w355) -> ()
          n245 = global write "全局 数据数组大小.vi" "数据数组大小"(w356) -> ()
        }
      }
    }
    frame "3021" {
      n246 = call "设置仪器参数命令解析.vi"("String输入"=w368) -> ("设置参数信息数组"=w369:string[][])  [unwired: 9 in, 1 out]
      n247 = for {
        tunnel: w369 -> [w372] mode=indexing
        # "同时设置几个参数?"
        n248 = flat-sequence {
          tunnel: w372 -> [w382]
          tunnel: [w373] -> w370
          tunnel: [w434] -> w371
          tunnel: w370 -> [w434]
          tunnel: w371 -> [w438]
          frame #0 {
            # "设置仪表参数"
            # "3|4个字节"
            # "反控指令"
            # "发命令给中控"
            # "1.因子编码\n2.关键参数\n3.值"
            n249 = Index Array(array=w382) -> (element #1=w381:string, element #2=w378:string, element #3=w377:string)  [unwired: 3 in]
            n250 = case shown="\"w01001\"" w381 {
              tunnel: [u16 0 ("starting address") u16 1 ("starting address") u16 2 ("starting address") u16 3 ("starting address") u16 4 ("starting address") u16 5 ("starting address") u16 6 ("starting address") u16 7 ("starting address") u16 8 ("starting address") u16 9 ("starting address") u16 10 ("starting address") u16 11 ("starting address") u16 12 ("starting address") u16 13 ("starting address")] -> w376
              frame "", Default {
              }
              frame "w01019" {
              }
              frame "w01001" {
              }
              frame "w21003" {
              }
              frame "w21001" {
              }
              frame "w21011" {
              }
              frame "w01018" {
              }
              frame "w01014" {
              }
              frame "w01010" {
              }
              frame "w01009" {
              }
              frame "w01003" {
              }
              frame "w01016" {
              }
              frame "w19011" {
              }
              frame "w01100" {
              }
            }
            n251 = case shown="\"i13101\"" w378 {
              tunnel: [u16 256 ("starting address") u16 256 ("starting address") u16 260 ("starting address") u16 264 ("starting address") u16 268 ("starting address") u16 272 ("starting address") u16 276 ("starting address") u16 280 ("starting address") u16 284 ("starting address") u16 288 ("starting address") u16 292 ("starting address") u16 296 ("starting address") u16 300 ("starting address") u16 304 ("starting address") u16 308 ("starting address") u16 312 ("starting address") u16 316 ("starting address") u16 320 ("starting address") u16 356 ("starting address") u16 360 ("starting address") u16 364 ("starting address") u16 368 ("starting address") u16 372 ("starting address") u16 376 ("starting address") u16 380 ("starting address") u16 384 ("starting address") u16 388 ("starting address") u16 392 ("starting address")] -> w373
              frame "", Default {
              }
              frame "i13001" {
              }
              frame "i13002" {
              }
              frame "i13003" {
              }
              frame "i13004" {
              }
              frame "i13005" {
              }
              frame "i13006" {
              }
              frame "i13007" {
              }
              frame "i13008" {
              }
              frame "i13009" {
              }
              frame "i13010" {
              }
              frame "i13011" {
              }
              frame "i13012" {
              }
              frame "i13013" {
              }
              frame "i13014" {
              }
              frame "i13015" {
              }
              frame "i13016" {
              }
              frame "i13017" {
              }
              frame "i13101" {
              }
              frame "i13102" {
              }
              frame "i13103" {
              }
              frame "i13104" {
              }
              frame "i13105" {
              }
              frame "i13106" {
              }
              frame "i13107" {
              }
              frame "i13108" {
              }
              frame "i13109" {
              }
              frame "i13110" {
              }
            }
            n252 = case shown="\"i13006\", \"i13013\"" w378 {
              tunnel: w377 -> [w386 w391]
              tunnel: [w384 w387] -> w375
              frame "假", Default {
                n253 = Fract/Exp String To Number(string=w386) -> (number=w383:dbl)  [unwired: 3 in, 1 out]
                n254 = Build Array(w383) -> (w385:dbl[])
                n255 = call "FloatToHex.vi"("浮点数"=w385) -> ("DCBA整形输出"=w384:u16[])  [unwired: 10 in]
              }
              frame "i13006", "i13013" {
                n256 = call "格式时间字符串.vi"("字符串"=w391) -> ("连接的字符串"=w390:string)  [unwired: 10 in]
                n257 = call "日期字符串格式至时间格式转换(子VI).vi"("data[0]"=w390) -> ("time stamp"=w389:timestamp)  [unwired: 10 in]
                n258 = Build Array(w389) -> (w388:timestamp[])
                n259 = call "DateToHex.vi"("DATE"=w388) -> ("数组"=w387:u16[])  [unwired: 10 in]
              }
            }
            n260 = Build Array (concatenate)(w376, w375) -> (w374:u16[])
            n261 = call "Modbus Master.vi"("starting address"=w373, "holding register values"=w374, "读取写入选择"="写入", "Unit ID"=u8 1) -> ()  [unwired: 5 in, 7 out]
          }
          frame #1 {
            n262 = Wait (ms)(milliseconds to wait=u32 2000 ("等待时间（毫秒）")) -> ()  [unwired: 1 out]
          }
          frame #2 {
            n263 = global write "全局1.vi" "table元素"("反控命令" ("新元素/子数组")) -> ()
            n264 = call "Modbus Master.vi"("starting address"=w438, "holding register values"=u16[] [0], "读取写入选择"="写入", "Unit ID"=u8 1) -> ()  [unwired: 5 in, 7 out]
          }
        }
      }
    }
    frame "3040" {
      n265 = global write "全局1.vi" "table元素"("提取现场系统信息" ("新元素/子数组")) -> ()
    }
    frame "3041" {
      n266 = call "数据表比对.vi"("table输入"="环境参数" ("新元素/子数组")) -> ("columns输出"=w442:string[], "待发送数据"=w444:string[][])  [unwired: 7 in, 2 out]
      n267 = global write "全局 环境参数.vi" "环境参数"(w444) -> ()
      n268 = global write "全局 环境参数.vi" "columns输出"(w442) -> ()
      n269 = global write "全局1.vi" "table元素"("提取经纬度环境信息" ("新元素/子数组")) -> ()
    }
    frame "3042" {
      # "反控指令"
      # "反控指令\n切换运行模式"
      # "发命令给中控"
      # "0维护，1常规，2应急，3质控"
      n270 = global write "全局1.vi" "table元素"("反控命令" ("新元素/子数组")) -> ()
      n271 = Search/Split String(string=w460, search string/char (-)="RunMode" ("搜索字符串/字符(-)")) -> (match + rest of string=w457:string)  [unwired: 1 in, 2 out]
      n272 = String Subset(string=w457, offset (0)=8 ("偏移量(0)"), length (rest)=1 ("长度（剩余）")) -> (substring=w447:string)
      n273 = Decimal String To Number(string=w447) -> (number=w446:i32)  [unwired: 2 in, 1 out]
      n274 = Insert Into Array(array=u16[] [] ("holding register values"), index=0 ("索引"), new element=w446) -> (w452:u16[])
      n275 = call "Modbus Master.vi"("starting address"=u16 0, "holding register values"=w452, "读取写入选择"="写入", "Unit ID"=u8 1) -> ()  [unwired: 5 in, 7 out]
    }
    frame "3043" {
      n276 = flat-sequence {
        frame #0 {
          n277 = global write "全局1.vi" "table元素"("反控命令" ("新元素/子数组")) -> ()
        }
        frame #1 {
          n278 = call <vilib>:"System Exec.vi"("command line"="cmd /c shutdown/r") -> ("error out"=w462:errorcluster)  [unwired: 7 in, 3 out]
          n279 = call <vilib>:"Clear Errors.vi"("error in (no error)"=w462) -> ()  [unwired: 5 in, 2 out]
        }
      }
    }
    frame "3044" {
      n280 = flat-sequence {
        frame #0 {
          # "反控指令"
          # "发命令给中控"
          n281 = call "Modbus Master.vi"("starting address"=u16 2, "holding register values"=u16[] [1], "读取写入选择"="写入", "Unit ID"=u8 1) -> ()  [unwired: 5 in, 7 out]
        }
        frame #1 {
          # "反控指令\n单次测量"
          n282 = Wait (ms)(milliseconds to wait=u32 2000 ("等待时间（毫秒）")) -> ()  [unwired: 1 out]
        }
        frame #2 {
          n283 = global write "全局1.vi" "table元素"("反控命令" ("新元素/子数组")) -> ()
          n284 = call "Modbus Master.vi"("starting address"=u16 2, "holding register values"=u16[] [0], "读取写入选择"="写入", "Unit ID"=u8 1) -> ()  [unwired: 5 in, 7 out]
        }
      }
    }
    frame "3045", "3046" {
      n285 = flat-sequence {
        frame #0 {
          # "发命令给中控"
          n286 = call "Modbus Master.vi"("starting address"=u16 3, "holding register values"=u16[] [1], "读取写入选择"="写入", "Unit ID"=u8 1) -> ()  [unwired: 5 in, 7 out]
        }
        frame #1 {
          # "反控指令"
          # "反控指令\n急停"
          # "3045"
          n287 = Wait (ms)(milliseconds to wait=u32 2000 ("等待时间（毫秒）")) -> ()  [unwired: 1 out]
        }
        frame #2 {
          n288 = global write "全局1.vi" "table元素"("反控命令" ("新元素/子数组")) -> ()
          n289 = call "Modbus Master.vi"("starting address"=u16 3, "holding register values"=u16[] [0], "读取写入选择"="写入", "Unit ID"=u8 1) -> ()  [unwired: 5 in, 7 out]
        }
      }
    }
    frame "3048" {
      # "启动全面清洗"
      n290 = flat-sequence {
        tunnel: [w486] -> w484
        tunnel: [w490] -> w485
        tunnel: w484 -> [w490]
        tunnel: w485 -> [w492]
        frame #0 {
          w486 = u16 8 ("starting address")
          # "发命令给中控"
          n291 = call "Modbus Master.vi"("starting address"=w486, "holding register values"=u16[] [1], "读取写入选择"="写入", "Unit ID"=u8 1) -> ()  [unwired: 5 in, 7 out]
        }
        frame #1 {
          n292 = Wait (ms)(milliseconds to wait=u32 2000 ("等待时间（毫秒）")) -> ()  [unwired: 1 out]
        }
        frame #2 {
          n293 = global write "全局1.vi" "table元素"("反控命令" ("新元素/子数组")) -> ()
          n294 = call "Modbus Master.vi"("starting address"=w492, "holding register values"=u16[] [0], "读取写入选择"="写入", "Unit ID"=u8 1) -> ()  [unwired: 5 in, 7 out]
        }
      }
    }
    frame "3056" {
      # "发回给平台"
      # "设置测量时间间隔"
      # "发命令给中控"
      n295 = global write "全局1.vi" "table元素"("反控命令" ("新元素/子数组")) -> ()
      n296 = Search/Split String(string=w508, search string/char (-)="RunInterval" ("搜索字符串/字符(-)")) -> (match + rest of string=w504:string)  [unwired: 1 in, 2 out]
      n297 = Decimal String To Number(string=w504, offset=12 ("偏移量(0)")) -> (number=w500:i32)  [unwired: 1 in, 1 out]
      n298 = Insert Into Array(array=u16[] [] ("holding register values"), index=0 ("索引"), new element=w500) -> (w499:u16[])
      n299 = call "Modbus Master.vi"("starting address"=u16 14, "holding register values"=w499, "读取写入选择"="写入", "Unit ID"=u8 1) -> ()  [unwired: 5 in, 7 out]
    }
    frame "3080", "3081", "3082", "3083", "3084", "3085", "3086" {
      n300 = flat-sequence {
        tunnel: w509 -> [w529]
        tunnel: [w527] -> w512
        tunnel: w510 -> [w525]
        tunnel: w512 -> [w554]
        tunnel: [w554] -> w511
        tunnel: w511 -> [w559]
        tunnel: [w556] -> _
        frame #0 {
          # "30 启动标液核查  1CODmn  2 氨氮  3总磷  4总氮  5CODCr\n31 加标回收\n32 平行样测试\n33 零点核查\n34 跨度核查\n35 校零\n36 校标"
          # "1CODmn  2 氨氮  3总磷  4总氮  5CODCr"
          # "启动单台仪器标液核查"
          # "发命令给中控"
          n301 = case shown="\"3081\"" w529 {
            tunnel: [u16 99 ("starting address") u16 30 ("starting address") u16 31 ("starting address") u16 32 ("starting address") u16 33 ("starting address") u16 34 ("starting address") u16 35 ("starting address") u16 36 ("starting address")] -> w527
            frame "", Default {
            }
            frame "3080" {
            }
            frame "3081" {
            }
            frame "3082" {
            }
            frame "3083" {
            }
            frame "3084" {
            }
            frame "3085" {
            }
            frame "3086" {
            }
          }
          n302 = Search/Split String(string=w525, search string/char (-)="PolId" ("搜索字符串/字符(-)")) -> (match + rest of string=w534:string)  [unwired: 1 in, 2 out]
          n303 = Search/Split String(string=w525, search string/char (-)="Volume" ("搜索字符串/字符(-)")) -> (match + rest of string=w522:string)  [unwired: 1 in, 2 out]
          n304 = String Subset(string=w534, offset (0)=6 ("偏移量(0)"), length (rest)=6 ("长度（剩余）")) -> (substring=w531:string)
          n305 = String Subset(string=w522, offset (0)=7 ("偏移量(0)"), length (rest)=8 ("长度（剩余）")) -> (substring=w521:string)
          n306 = case shown="\"w01019\"" w531 {
            tunnel: [0 ("长度（剩余）") 1 ("长度（剩余）") 2 ("长度（剩余）") 3 ("长度（剩余）") 4 ("长度（剩余）") 5 ("长度（剩余）")] -> w530
            frame "", Default {
            }
            frame "w01019" {
            }
            frame "w21003" {
            }
            frame "w21011" {
            }
            frame "w21001" {
            }
            frame "w01018" {
            }
          }
          n307 = Fract/Exp String To Number(string=w521) -> (number=w516:dbl)  [unwired: 3 in, 1 out]
          n308 = Build Array(w516) -> (w515:dbl[])
          n309 = call "FloatToHex.vi"("浮点数"=w515) -> ("DCBA整形输出"=w514:u16[])  [unwired: 10 in]
          n310 = call "Modbus Master.vi"("starting address"=u16 15, "holding register values"=w514, "读取写入选择"="写入", "Unit ID"=u8 1) -> ("error out"=w518:errorcluster)  [unwired: 5 in, 6 out]
          n311 = Insert Into Array(array=u16[] [] ("holding register values"), index=0 ("索引"), new element=w530) -> (w535:u16[])
          n312 = call "Modbus Master.vi"("starting address"=w527, "error in"=w518, "holding register values"=w535, "读取写入选择"="写入", "Unit ID"=u8 1) -> ()  [unwired: 4 in, 7 out]
        }
        frame #1 {
          n313 = Wait (ms)(milliseconds to wait=u32 2000 ("等待时间（毫秒）")) -> ()  [unwired: 1 out]
        }
        frame #2 {
          n314 = global write "全局1.vi" "table元素"("反控命令" ("新元素/子数组")) -> ()
          n315 = call "Modbus Master.vi"("starting address"=w559, "holding register values"=u16[] [0], "读取写入选择"="写入", "Unit ID"=u8 1) -> ("error out"=w556:errorcluster)  [unwired: 5 in, 6 out]
        }
      }
    }
    frame "3100" {
      # "获取软件版本号"
      n316 = global read "断电保存全局.vi" "应用环境"() -> (w563:T1)
      n317 = case shown="\"婉仪平台\"" w563 {
        tunnel: ["反控命令" ("新元素/子数组") "反控命令" ("新元素/子数组") "获取软件版本号" ("新元素/子数组")] -> w562
        frame "STD", Default {
        }
        frame "GB212" {
        }
        frame "婉仪平台" {
        }
      }
      n318 = global write "全局1.vi" "table元素"(w562) -> ()
    }
    frame "3101" {
      # "软件升级"
      n319 = global read "断电保存全局.vi" "应用环境"() -> (w573:T1)
      n320 = Search/Split String(string=w571, search string/char (-)="URL=" ("搜索字符串/字符(-)")) -> (match + rest of string=w569:string)  [unwired: 1 in, 2 out]
      n321 = case shown="\"婉仪平台\"" w573 {
        tunnel: ["反控命令" ("新元素/子数组") "反控命令" ("新元素/子数组") "反控命令" ("新元素/子数组")] -> w572
        frame "STD", Default {
        }
        frame "GB212" {
        }
        frame "婉仪平台" {
          n322 = flat-sequence {
            tunnel: [w580] -> w578
            tunnel: [w584] -> w577
            tunnel: w578 -> [w584]
            tunnel: w577 -> [w587]
            tunnel: [w586] -> w576
            frame #0 {
              w580 = u16 858 ("starting address")
              n323 = call "Modbus Master.vi"("starting address"=w580, "holding register values"=u16[] [1], "读取写入选择"="写入", "Unit ID"=u8 1) -> ()  [unwired: 5 in, 7 out]
            }
            frame #1 {
              n324 = Wait (ms)(milliseconds to wait=u32 2000 ("等待时间（毫秒）")) -> ()  [unwired: 1 out]
            }
            frame #2 {
              n325 = call "Modbus Master.vi"("starting address"=w587, "holding register values"=u16[] [0], "读取写入选择"="写入", "Unit ID"=u8 1) -> ("error out"=w586:errorcluster)  [unwired: 5 in, 6 out]
            }
          }
          n326 = case shown="无错误" w576 {
            frame No Error {
              n327 = call "autoupdate.vi"() -> ()  [unwired: 12 in]
            }
            frame Error {
            }
          }
        }
      }
      n328 = Bundle("数据"=w569) -> (w568:cluster{"数据":string})  [unwired: 1 in]
      n329 = call "添加URL.vi"("URL"="URL", "簇"=w568) -> ()  [unwired: 8 in, 2 out]
      n330 = global write "全局1.vi" "table元素"(w572) -> ()
    }
    frame "3102" {
      # "获取固件版本号"
      n331 = global read "断电保存全局.vi" "应用环境"() -> (w599:T1)
      n332 = Search/Split String(string=w592, search string/char (-)="PolId" ("搜索字符串/字符(-)")) -> (match + rest of string=w594:string)  [unwired: 1 in, 2 out]
      n333 = case shown="\"婉仪平台\"" w599 {
        tunnel: ["反控命令" ("新元素/子数组") "反控命令" ("新元素/子数组") "获取仪器软件版本号" ("新元素/子数组")] -> w598
        frame "STD", Default {
        }
        frame "GB212" {
        }
        frame "婉仪平台" {
        }
      }
      n334 = String Subset(string=w594, offset (0)=6 ("偏移量(0)"), length (rest)=6 ("长度（剩余）")) -> (substring=w597:string)
      n335 = case shown="\"w01018\"" w597 {
        tunnel: [0 ("长度（剩余）") 1 ("长度（剩余）") 2 ("长度（剩余）") 3 ("长度（剩余）") 4 ("长度（剩余）") 5 ("长度（剩余）")] -> w591
        frame "", Default {
        }
        frame "w01019" {
        }
        frame "w21003" {
        }
        frame "w21011" {
        }
        frame "w21001" {
        }
        frame "w01018" {
        }
      }
      n336 = global write "全局 小时数据发送次数.vi" "小时数据发送次数"(w591) -> ()
      n337 = global write "全局1.vi" "table元素"(w598) -> ()
    }
    frame "3103" {
      # "固件升级"
      n338 = Search/Split String(string=w613, search string/char (-)="PolId" ("搜索字符串/字符(-)")) -> (match + rest of string=w616:string)  [unwired: 1 in, 2 out]
      n339 = Search/Split String(string=w613, search string/char (-)="URL=" ("搜索字符串/字符(-)")) -> (match + rest of string=w619:string)  [unwired: 1 in, 2 out]
      n340 = String Subset(string=w616, offset (0)=6 ("偏移量(0)"), length (rest)=6 ("长度（剩余）")) -> (substring=w610:string)
      n341 = case shown="\"w21003\"" w610 {
        tunnel: [0 ("长度（剩余）") 1 ("长度（剩余）") 2 ("长度（剩余）") 3 ("长度（剩余）") 4 ("长度（剩余）") 5 ("长度（剩余）")] -> w609
        frame "", Default {
        }
        frame "w01019" {
        }
        frame "w21003" {
        }
        frame "w21011" {
        }
        frame "w21001" {
        }
        frame "w01018" {
        }
      }
      n342 = Concatenate Strings(w610, "URL" ("URL")) -> (w611:string)
      n343 = Bundle("数据"=w619) -> (w618:cluster{"数据":string})  [unwired: 1 in]
      n344 = global read "断电保存全局.vi" "应用环境"() -> (w622:T1)
      n345 = call "添加URL.vi"("URL"=w611, "簇"=w618) -> ()  [unwired: 8 in, 2 out]
      n346 = case shown="\"婉仪平台\"" w622 {
        tunnel: ["反控命令" ("新元素/子数组") "反控命令" ("新元素/子数组") "反控命令" ("新元素/子数组")] -> w621
        tunnel: w609 -> [_ _ w631]
        frame "STD", Default {
        }
        frame "GB212" {
        }
        frame "婉仪平台" {
          n347 = flat-sequence {
            tunnel: [w638] -> w634
            tunnel: w631 -> [w637]
            tunnel: [w641] -> w633
            tunnel: w634 -> [w641]
            tunnel: w633 -> [w644]
            tunnel: [w643] -> w632
            frame #0 {
              w638 = u16 866 ("starting address")
              n348 = Build Array(w637) -> (w636:i32[])
              n349 = call "Modbus Master.vi"("starting address"=w638, "holding register values"=w636, "读取写入选择"="写入", "Unit ID"=u8 1) -> ()  [unwired: 5 in, 7 out]
            }
            frame #1 {
              n350 = Wait (ms)(milliseconds to wait=u32 2000 ("等待时间（毫秒）")) -> ()  [unwired: 1 out]
            }
            frame #2 {
              n351 = call "Modbus Master.vi"("starting address"=w644, "holding register values"=u16[] [0], "读取写入选择"="写入", "Unit ID"=u8 1) -> ("error out"=w643:errorcluster)  [unwired: 5 in, 6 out]
            }
          }
          n352 = case shown="无错误" w632 {
            frame No Error {
              n353 = call "autoupdate.vi"() -> ()  [unwired: 12 in]
            }
            frame Error {
            }
          }
        }
      }
      n354 = global write "全局1.vi" "table元素"(w621) -> ()
    }
    frame "3200" {
      # "启动剖面水样测试/仪表做样"
      n355 = global read "断电保存全局.vi" "应用环境"() -> (w650:T1)
      n356 = case shown="\"婉仪平台\"" w650 {
        tunnel: w649 -> [_ w662]
        tunnel: w648 -> [_ w661]
        frame "STD", Default {
          n357 = flat-sequence {
            frame #0 {
              # "反控指令"
              # "发命令给中控"
              n358 = call "Modbus Master.vi"("starting address"=u16 6, "holding register values"=u16[] [1], "读取写入选择"="写入", "Unit ID"=u8 1) -> ()  [unwired: 5 in, 7 out]
            }
            frame #1 {
              # "反控指令\n单次测量"
              n359 = Wait (ms)(milliseconds to wait=u32 2000 ("等待时间（毫秒）")) -> ()  [unwired: 1 out]
            }
            frame #2 {
              n360 = global write "全局1.vi" "table元素"("反控命令" ("新元素/子数组")) -> ()
              n361 = call "Modbus Master.vi"("starting address"=u16 6, "holding register values"=u16[] [0], "读取写入选择"="写入", "Unit ID"=u8 1) -> ()  [unwired: 5 in, 7 out]
            }
          }
        }
        frame "婉仪平台" {
          n362 = flat-sequence {
            tunnel: w662 -> [_]
            tunnel: [w666] -> w664
            tunnel: w661 -> [w665]
            tunnel: w664 -> [w684]
            tunnel: [w684] -> w663
            tunnel: w663 -> [w689]
            tunnel: [w686] -> _
            frame #0 {
              w666 = u16 37 ("starting address")
              # "30 启动标液核查  1CODmn  2 氨氮  3总磷  4总氮  5CODCr\n31 加标回收\n32 平行样测试\n33 零点核查\n34 跨度核查\n35 校零\n36 校标"
              # "1CODmn  2 氨氮  3总磷  4总氮  5CODCr"
              # "启动单台仪器标液核查"
              # "发命令给中控"
              n363 = Search/Split String(string=w665, search string/char (-)="PolId" ("搜索字符串/字符(-)")) -> (match + rest of string=w672:string)  [unwired: 1 in, 2 out]
              n364 = String Subset(string=w672, offset (0)=6 ("偏移量(0)"), length (rest)=6 ("长度（剩余）")) -> (substring=w669:string)
              n365 = case shown="\"w01019\"" w669 {
                tunnel: [0 ("长度（剩余）") 1 ("长度（剩余）") 2 ("长度（剩余）") 3 ("长度（剩余）") 4 ("长度（剩余）") 5 ("长度（剩余）")] -> w668
                frame "", Default {
                }
                frame "w01019" {
                }
                frame "w21003" {
                }
                frame "w21011" {
                }
                frame "w21001" {
                }
                frame "w01018" {
                }
              }
              n366 = Insert Into Array(array=u16[] [] ("holding register values"), index=0 ("索引"), new element=w668) -> (w673:u16[])
              n367 = call "Modbus Master.vi"("starting address"=w666, "holding register values"=w673, "读取写入选择"="写入", "Unit ID"=u8 1) -> ()  [unwired: 5 in, 7 out]
            }
            frame #1 {
              n368 = Wait (ms)(milliseconds to wait=u32 2000 ("等待时间（毫秒）")) -> ()  [unwired: 1 out]
            }
            frame #2 {
              n369 = global write "全局1.vi" "table元素"("反控命令" ("新元素/子数组")) -> ()
              n370 = call "Modbus Master.vi"("starting address"=w689, "holding register values"=u16[] [0], "读取写入选择"="写入", "Unit ID"=u8 1) -> ("error out"=w686:errorcluster)  [unwired: 5 in, 6 out]
            }
          }
        }
      }
    }
    frame "3201" {
      # "开启摄像头电源"
      n371 = flat-sequence {
        frame #0 {
          # "反控指令"
          # "发命令给中控"
          n372 = call "Modbus Master.vi"("starting address"=u16 7, "holding register values"=u16[] [1], "读取写入选择"="写入", "Unit ID"=u8 1) -> ()  [unwired: 5 in, 7 out]
        }
        frame #1 {
          # "反控指令\n单次测量"
          n373 = Wait (ms)(milliseconds to wait=u32 2000 ("等待时间（毫秒）")) -> ()  [unwired: 1 out]
        }
        frame #2 {
          n374 = global write "全局1.vi" "table元素"("反控命令" ("新元素/子数组")) -> ()
          n375 = call "Modbus Master.vi"("starting address"=u16 7, "holding register values"=u16[] [0], "读取写入选择"="写入", "Unit ID"=u8 1) -> ()  [unwired: 5 in, 7 out]
        }
      }
    }
  }
  "反控命令错误？" <- w2
  n376 = case shown="假" w2 {
    tunnel: w1 -> [w702 _]
    frame False {
      n377 = global write "全局 反控命令枚举.vi" "是否判断反馈？"(w702) -> ()
    }
    frame True {
    }
  }
